vi "boolean.vi"() -> ()   [LabVIEW 2020]
panel:
  out "output":bool
  in  "input":bool
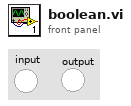
[diagram p1: front panel]
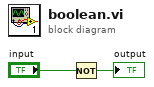
[diagram p0: block diagram]
diagram:
  n1 = Not(x="input") -> (.not. x?=→"output":bool)
